vi "TDMSmanager.vi"(8 "ErrorIn":errorcluster, 11 "QueuesIn":T1) -> (0 "ErrorOut":errorcluster, 3 "QueuesOut":T1)   [LabVIEW 2019]
uses:
  utilities/AQueues.ctl
  AmasterVIs/ACommand.ctl
  analyzeAccelerationDataVIs/AccelerationDataFrames.ctl
  analyzeAccelerationDataVIs/AnalyzedVibrationsData.ctl
  analyzeAccelerationDataVIs/calculateFaultIndicatorsVIs/FaultDetections.ctl
  analyzeAccelerationDataVIs/calculateFaultIndicatorsVIs/ParameterFaultDetection.ctl
  analyzeAccelerationDataVIs/calculateFaultIndicatorsVIs/FaultParameter.ctl
  analyzeAccelerationDataVIs/calculateFaultIndicatorsVIs/FrequencyFaultDetection.ctl
  analyzeAccelerationDataVIs/calculateFaultIndicatorsVIs/OrdersFaultDetection.ctl
  TDMSmanagerVIs/TDMSAnalyzerData.ctl
  TDMSmanagerVIs/TDMSAnalyzerDataType.ctl
  TDMSmanagerVIs/TDMSmanagerState.ctl
  AmasterVIs/AThreads.ctl
  <vilib>/Platform/TimedLoop/XDataNode/timing_clust.ctl
  <vilib>/Platform/TimedLoop/XDataNode/nitl_modes.ctl
  <vilib>/Platform/TimedLoop/XDataNode/wakeup.ctl
  <vilib>/platform/TimedLoop/XDataNode/XDataNode.xnode
  <vilib>/Platform/TimedLoop/XDataNode/XDNodeRunTimeDep.lvlib
panel:
  in  "Restart":bool
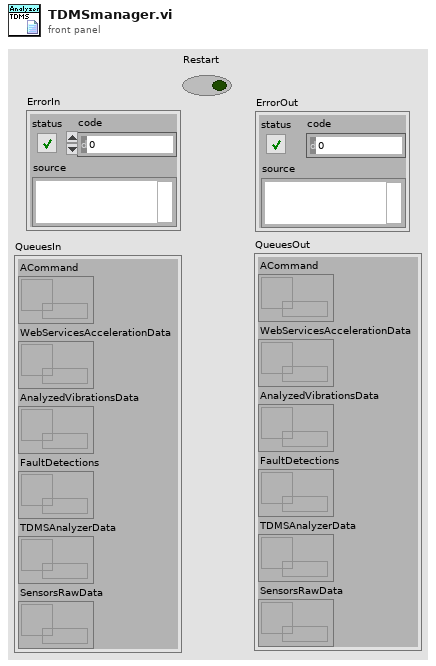
[diagram p1: front panel]
types:
  T1 = typedef "AQueues.ctl" = cluster{"ACommand":refnum<queue>, "WebServicesAccelerationData":refnum<queue>, "AnalyzedVibrationsData":refnum<queue>, "FaultDetections":refnum<queue>, "TDMSAnalyzerData":refnum<queue>, "SensorsRawData":refnum<queue>}
  T2 = typedef "AThreads.ctl" = enum16{"UI", "analyzeAccelerationData", "aquireAccelerationData", "communicateWebServices", "TDMSmanager", "aquireTachoSignal"}
  T3 = typedef "TDMSmanagerState.ctl" = enum16{"Idle", "SaveToFile", "SendFiles", "DeleteFiles", "CloseReference", "InitFileToSave"}
  T4 = typedef "XDNodeRunTimeDep.lvlib/timing_clust.ctl" = cluster{"Expected End [f-1]":u64, "Actual End [f-1]":u64, "Finished Late? [f-1]":bool, "Expected End [i-1]":u64, "Actual End [i-1]":u64, "Finished Late? [i-1]":bool, "Expected Start [i]":u64, "Actual Start [i]":u64, "Expected Start [f]":u64, "Actual Start [f]":u64, "Source Name":string, "Structure Name":string, "Period":i64, "Deadline":i64, "Offset":i64, "Start":i64, "Priority":i32, "Timeout":i32, "Mode":T5, "Wakeup Reason":T6, "Error":errorcluster, "Source Type":string, "Secondary Source Type":string, "Global End Time":u64, "Global Start Time":u64, "Frame Duration":u64, "Iteration Duration":u64, "Assigned CPU":i32, "I/O Scan Engine Mode":u32}
  T5 = typedef "XDNodeRunTimeDep.lvlib/nitl_modes.ctl" = enum32{"No Change", "Process missed periods, maintain original phase", "Discard missed periods, maintain original phase", "Process missed periods, ignore original phase", "Discard missed periods, ignore original phase"}
  T6 = typedef "XDNodeRunTimeDep.lvlib/wakeup.ctl" = enum32{"Normal", "Aborted", "Asynchronous wakeup", "Timing source error", "Timed loop error", "Timeout"}
  T7 = typedef "ACommand.ctl" = enum16{"None", "Start", "Stop", "Restart", "SendFilesData", "DeleteAllData"}
  T8 = enum16{"open", "replace", "create", "open or create", "replace or create", "replace or create with confirmation"}
  T9 = enum16{"open", "open or create", "create or replace", "create", "open (read-only)"}
  T10 = typedef "TDMSAnalyzerDataType.ctl" = enum16{"FileDataStart", "FileGroup", "FileDataStop", "NewFile", "EndOfFile"}
  T11 = typedef "TDMSAnalyzerData.ctl" = cluster{"TDMSAnalyzerDataType":T10, "group name out":string, "channel name(s) out":string[], "data":waveform(dbl)[], "File name":string}
  T12 = typedef "AnalyzerSettings.ctl" = cluster{"Create NS Timeout Code":i32, "Destroy NS Timeout Code":i32, "All threads":T2[], "AnalysisSettings":T13}
  T13 = typedef "AnalysisSettings.ctl" = cluster{"Fault Thresholds":T14, "Analysis series name":string, "Save data analysis?":bool, "Band size":i32, "OrderAnalysis?":bool, "Accelerometer":T16, "fs [Hz]":dbl, "Pulse per revolution":u16}
  T14 = typedef "Thresholds.ctl" = cluster{"Parameters labels":T15[], "Parameters thresholds":dbl[], "Freqs and thresholds":dbl[][], "Orders and thresholds":dbl[][]}
  T15 = typedef "FaultParameter.ctl" = enum16{"Kurtosis", "RMS", "Crest factor"}
  T16 = typedef "Accelerometer.ctl" = enum16{"None", "MPU6050", "MMA7351"}
  T17 = typedef "FaultDetections.ctl" = cluster{"Parameters fault detection":T18[], "Frequencies fault detection":T19[], "Orders fault detection":T20[]}
  T18 = typedef "ParameterFaultDetection.ctl" = cluster{"Axes Values":dbl[], "Axes Fault Detection":bool[], "Parameter Label":T15}
  T19 = typedef "FrequencyFaultDetection.ctl" = cluster{"Axes Values":dbl[], "Axes Fault Detection":bool[], "Frequency":dbl}
  T20 = typedef "OrdersFaultDetection.ctl" = cluster{"Order":dbl, "Axes Fault Detection":bool[], "Axes Values":dbl[]}
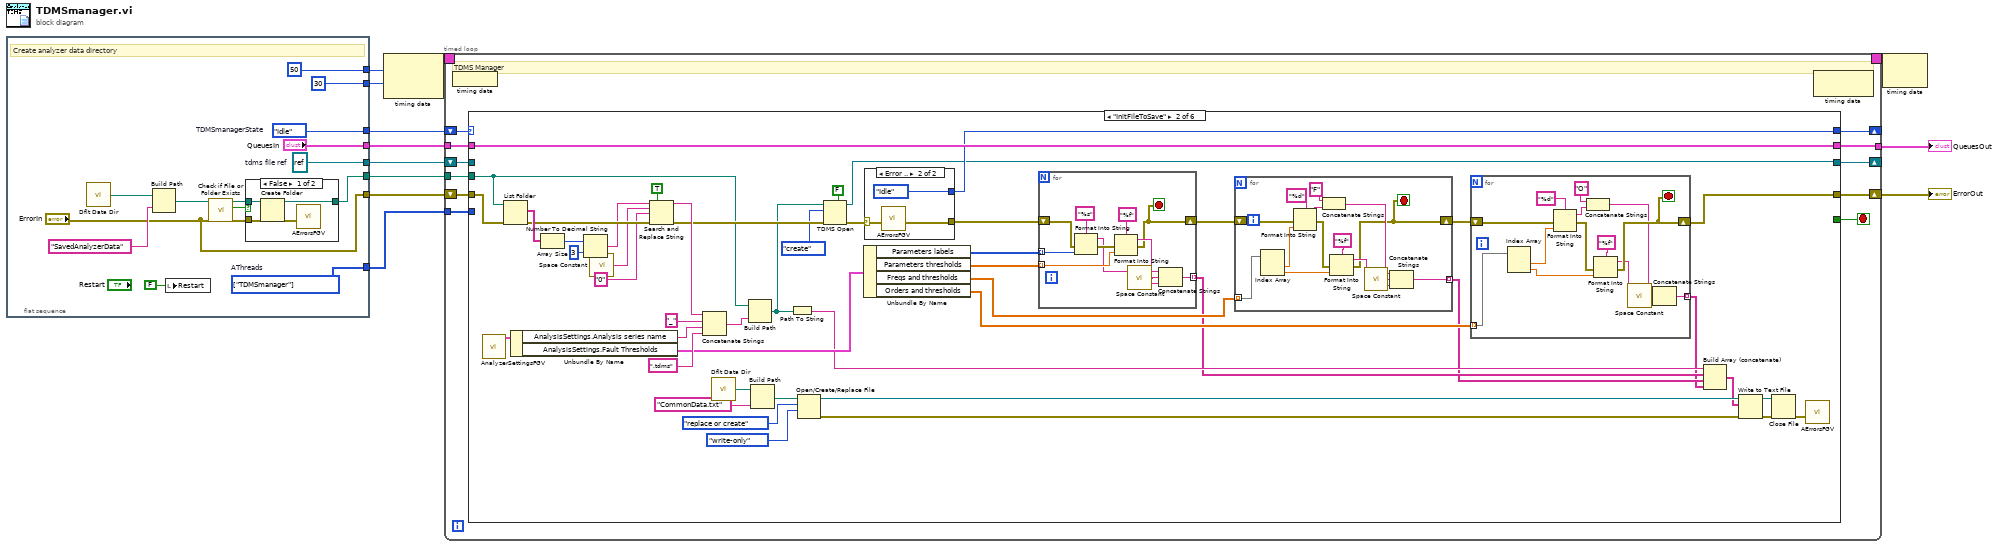
[diagram p0: block diagram]
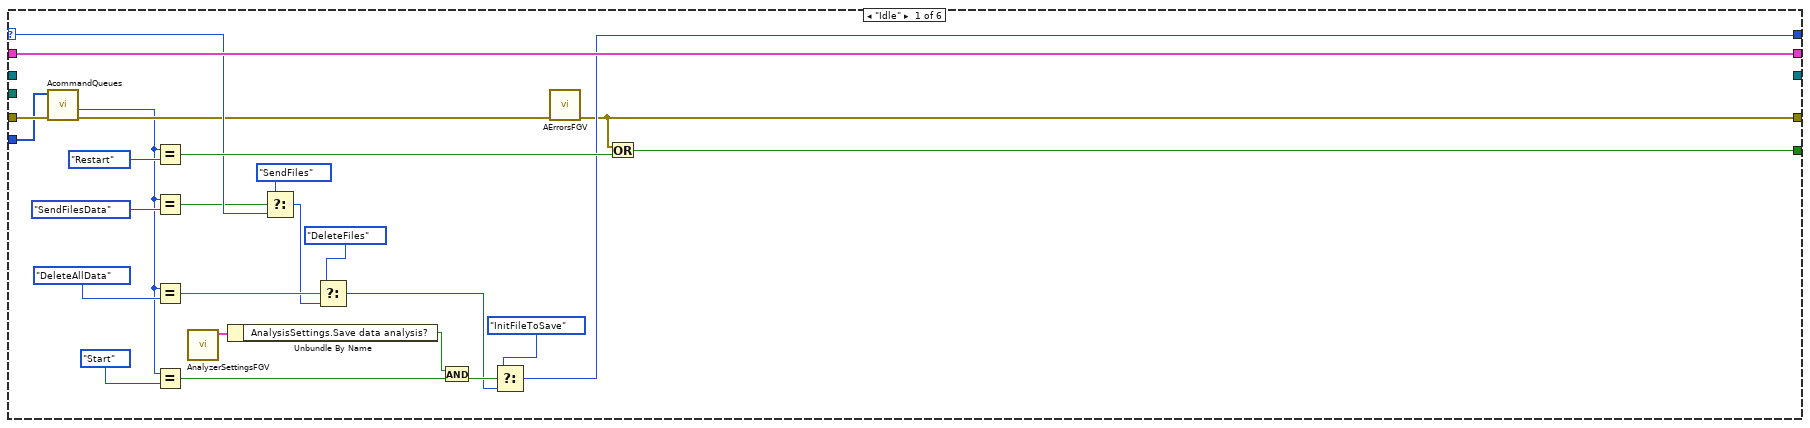
[diagram p2: hidden frame]
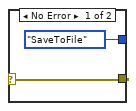
[diagram p3: hidden frame]
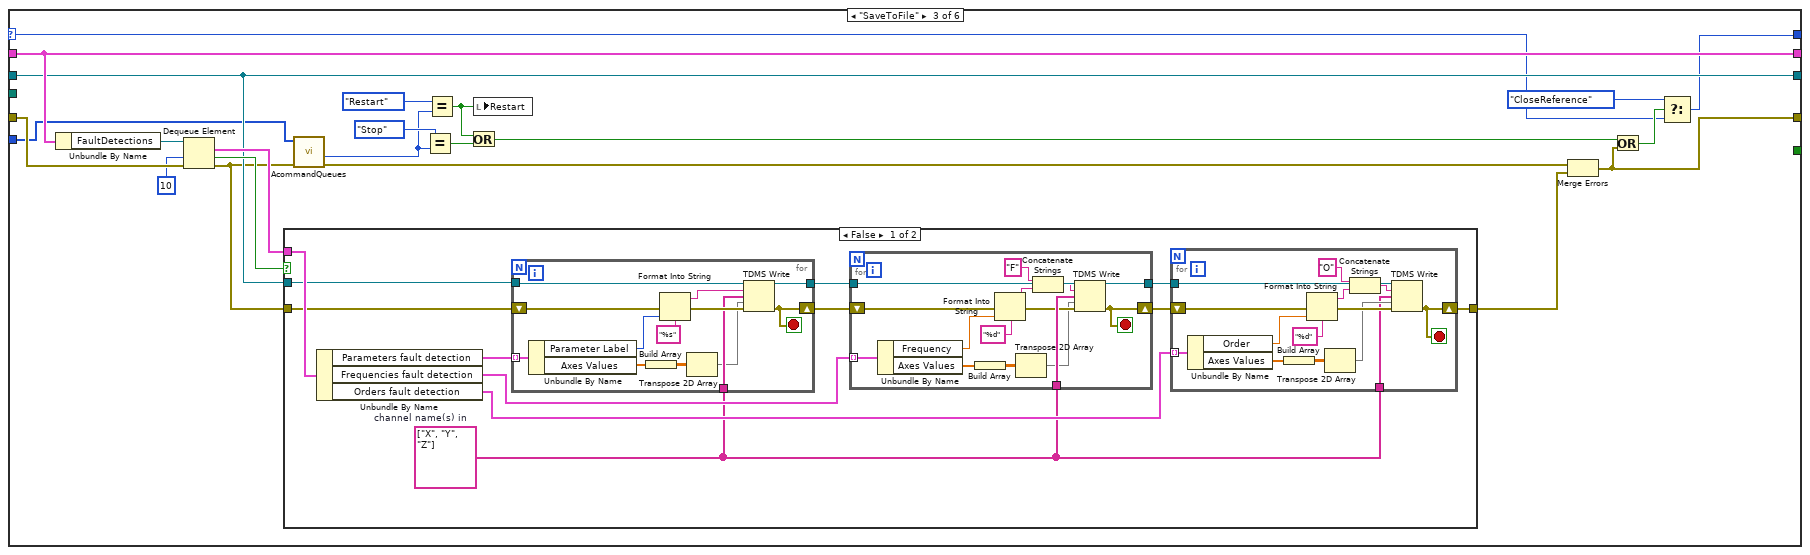
[diagram p4: hidden frame]
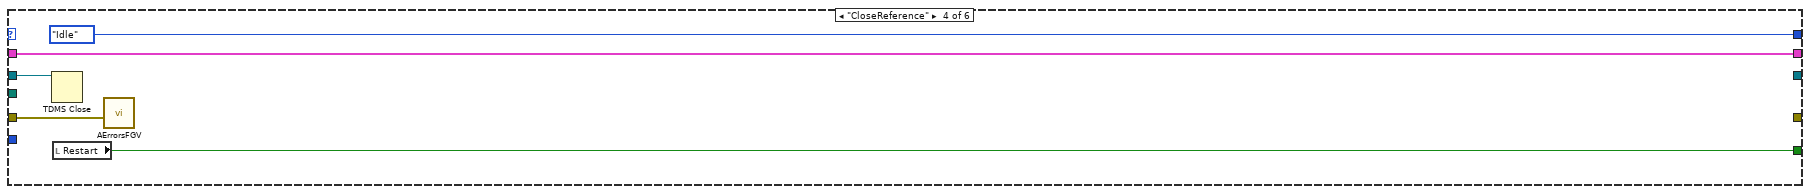
[diagram p6: hidden frame]
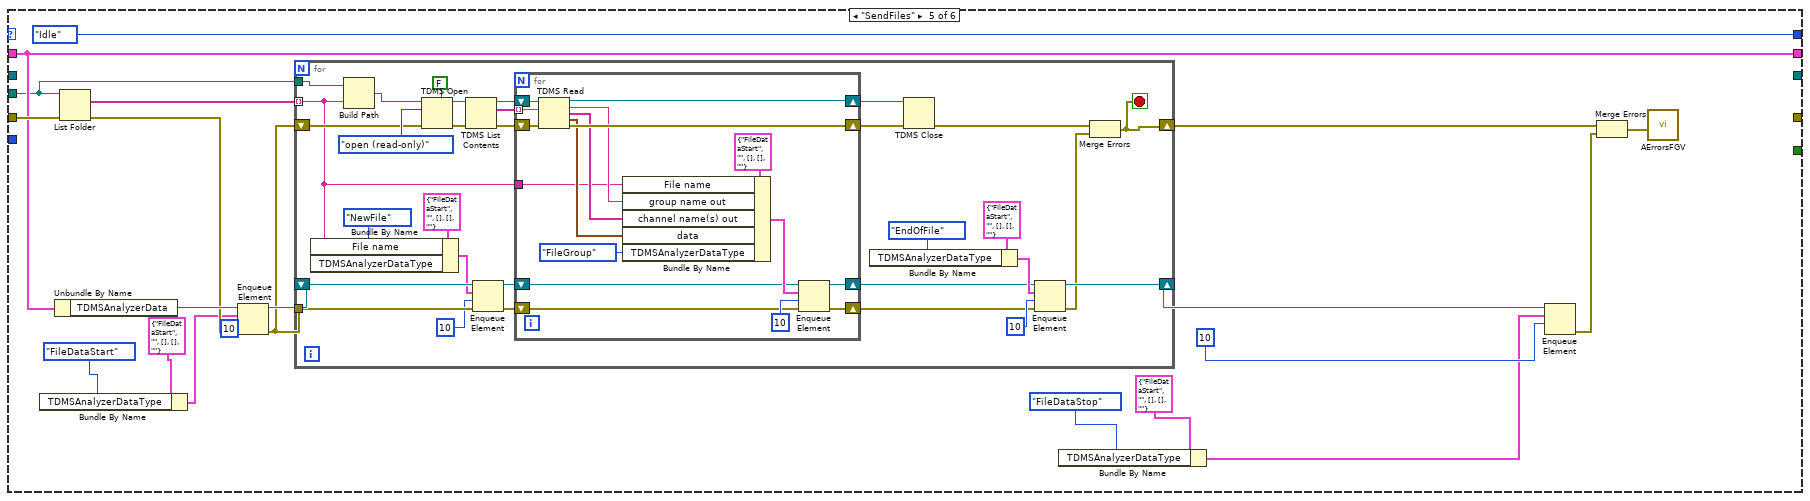
[diagram p7: hidden frame]
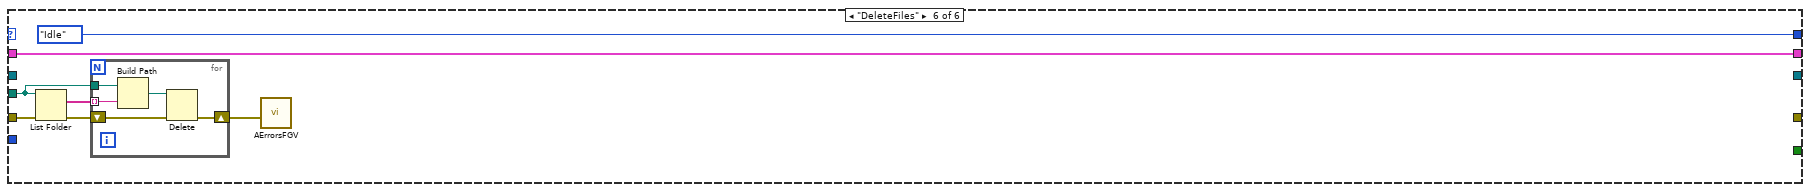
[diagram p8: hidden frame]
diagram:
  n1 = flat-sequence {
    tunnel: [w27] -> w12
    tunnel: ["QueuesIn"] -> w11
    tunnel: ["ErrorIn"] -> w8
    tunnel: [w20] -> w7
    tunnel: [w19] -> w6
    tunnel: [w17] -> w5
    tunnel: [i64 50 ("Period")] -> w2
    tunnel: [30 ("Priority")] -> w1
    frame #0 {
      w17 = T2[] [enum."TDMSmanager"] items=["UI", "analyzeAccelerationData", "aquireAccelerationData", "communicateWebServices", "TDMSmanager", "aquireTachoSignal"]  # AThreads
      w19 = refnum<k34> refnum  # tdms file ref
      w27 = TDMSmanagerState."Idle"  # TDMSmanagerState
      # "Create analyzer data directory"
      n2 = call <vilib>:"Dflt Data Dir.vi"() -> ("App:Default Data Directory"=w15:path)
      n3 = Build Path(base path=w15, name or relative path="SavedAnalyzerData") -> (appended path=w24:path)
      n4 = local write "Restart"(FALSE ("Restart")) -> ()
      n5 = call <vilib>:"Check if File or Folder Exists.vi"("error in (no error)"="ErrorIn", "path"=w24) -> ("error out"=w21:errorcluster, "file or folder exists?"=w23:bool, "dup path"=w22:path)  [unwired: 7 in]
      n6 = case shown="False" w23 {
        tunnel: w22 -> [w31 w32]
        tunnel: w21 -> [w28 _]
        tunnel: [w30 w32] -> w20
        frame False {
          n7 = Create Folder(path (use dialog)=w31, error in=w28) -> (created path=w30:path, error out=w29:errorcluster)  [unwired: 1 in, 1 out]
          n8 = call "AErrorsFGV.vi"("InternalErrorIn"=w29) -> ()  [unwired: 7 in, 4 out]
        }
        frame True {
        }
      }
    }
  }
  n9 = node-c288(w2, w1) -> (w4:T4)
  n10 = timed-loop {
    shift-right: [w40] -> _
    shift-left: w12 -> [w43]
    tunnel: w11 -> [w42]
    tunnel: [w41] -> w10
    shift-right: [w34] -> _
    shift-left: w6 -> [w36]
    shift-right: [w38] -> w9
    shift-left: w8 -> [w39]
    tunnel: w7 -> [w35]
    tunnel: w5 -> [w33]
    timing: w4 -> [_]
    timing-out: [_] -> w3
    stop <- w37 stop-if-true
    # "TDMS Manager"
    n11 = node-c288() -> ()  [unwired: 1 in]
    n12 = case shown="\"InitFileToSave\"" w43 {
      selector: w43 -> [w59 _ w169 _ _ _]
      tunnel: w42 -> [w70 w118 w184 w241 w255 w319]
      tunnel: [w70 w118 w184 w241 w255 w319] -> w41
      tunnel: [w53 w103 w167 TDMSmanagerState."Idle" ("TDMSmanagerState") TDMSmanagerState."Idle" ("TDMSmanagerState") TDMSmanagerState."Idle" ("TDMSmanagerState")] -> w40
      tunnel: w39 -> [w49 w117 w182 w243 w265 w317]
      tunnel: [w50 w79 w172 _ _ _] -> w38
      tunnel: [w51 _ _ w240 _ _] -> w37
      tunnel: w36 -> [_ _ w178 w244 _ _]
      tunnel: w35 -> [_ w97 _ _ w246 w314]
      tunnel: [_ w76 w178 _ _ _] -> w34
      tunnel: w33 -> [w48 _ w163 _ _ _]
      frame "Idle" {
        n13 = call "AcommandQueues.vi"("ErrorIn"=w49, "AThreads"=w48) -> ("ErrorOut"=w47:errorcluster, "ACommandOut"=w46:T7)  [unwired: 8 in]
        n14 = Equal?(x=w46, y=ACommand."Restart") -> (x = y?=w65:bool)
        n15 = Equal?(x=w46, y=ACommand."SendFilesData") -> (x = y?=w58:bool)
        n16 = Equal?(x=w46, y=ACommand."DeleteAllData") -> (x = y?=w55:bool)
        n17 = Equal?(x=w46, y=ACommand."Start") -> (x = y?=w63:bool)
        n18 = call "AnalyzerSettingsFGV.vi"() -> ("GlobalSettingsOut"=w64:T12)  [unwired: 11 in]
        n19 = Unbundle By Name(w64) -> ("AnalysisSettings.Save data analysis?"=w61:bool)
        n20 = Select(t=TDMSmanagerState."SendFiles", s=w58, f=w59) -> (s? t:f=w54:T3)
        n21 = Select(t=TDMSmanagerState."DeleteFiles", s=w55, f=w54) -> (s? t:f=w52:T3)
        n22 = And(x=w61, y=w63) -> (x .and. y?=w62:bool)
        n23 = Select(t=TDMSmanagerState."InitFileToSave", s=w62, f=w52) -> (s? t:f=w53:T3)
        n24 = call "AErrorsFGV.vi"("CriticalErrorIn"=w47) -> ("CriticalErrorOut"=w50:errorcluster)  [unwired: 7 in, 3 out]
        n25 = Or(x=w50, y=w65) -> (x .or. y?=w51:bool)
      }
      frame "InitFileToSave" {
        n26 = call "AnalyzerSettingsFGV.vi"() -> ("GlobalSettingsOut"=w102:T12)  [unwired: 11 in]
        n27 = List Folder(path=w97, error in=w117) -> (filenames=w116:string[], error out=w113:errorcluster)  [unwired: 2 in, 2 out]
        n28 = Unbundle By Name(w102) -> ("AnalysisSettings.Analysis series name"=w100:string, "AnalysisSettings.Fault Thresholds"=w85:T14)
        n29 = Array Size(array=w116) -> (size(s)=w115:i32)
        n30 = Number To Decimal String(number=w115, width (-)=i16 3) -> (decimal integer string=w112:string)
        n31 = call <vilib>:"Space Constant.vi"() -> ("String"=w110:string)
        n32 = Search and Replace String(replace all?=TRUE ("replace all? (F)"), input string=w112, search string=w110, replace string="0" ("replace string (\"\")"), error in=w113) -> (result string=w108:string, error out=w107:errorcluster)  [unwired: 3 in, 2 out]
        n33 = Concatenate Strings(w108, "_" ("string"), w100, ".tdms" ("string")) -> (w91:string)
        n34 = call <vilib>:"Dflt Data Dir.vi"() -> ("App:Default Data Directory"=w89:path)
        n35 = Build Path(base path=w97, name or relative path=w91) -> (appended path=w88:path)
        n36 = Build Path(base path=w89, name or relative path="CommonData.txt") -> (appended path=w96:path)
        n37 = Path To String(path=w88) -> (string=w75:string)
        n38 = Open/Create/Replace File(file path (use dialog)=w96, operation (0:open)=T8."replace or create", access (0:read/write)=enum16{"read/write", "read-only", "write-only"}."write-only") -> (refnum out=w93:refnum<file>, error out=w92:errorcluster)  [unwired: 3 in, 1 out]
        n39 = TDMS Open(5:FALSE ("create index file? (T)"), 8:w107, 10:T9."create" ("operation (0:open)"), 11:w88) -> (0:w104:errorcluster, 3:w76:refnum<k34>)  [unwired: 3 in]
        n40 = Unbundle By Name(w85) -> ("Parameters labels"=w87:T15[], "Parameters thresholds"=w86:dbl[], "Freqs and thresholds"=w82:dbl[][], "Orders and thresholds"=w80:dbl[][])
        n41 = case shown="Error .." w104 {
          selector: w104 -> [w158 w161]
          tunnel: [TDMSmanagerState."SaveToFile" ("TDMSmanagerState") TDMSmanagerState."Idle" ("TDMSmanagerState")] -> w103
          tunnel: [w158 w160] -> w84
          frame No Error {
          }
          frame Error {
            n42 = call "AErrorsFGV.vi"("InternalErrorIn"=w161) -> ("InternalErrorOut"=w160:errorcluster)  [unwired: 7 in, 3 out]
          }
        }
        n43 = for {
          tunnel: w87 -> [w156] mode=indexing
          tunnel: w86 -> [w154] mode=indexing
          shift-right: [w147] -> w83
          shift-left: w84 -> [w155]
          tunnel: [w148] -> w74 mode=indexing
          stop <- w147 stop-if-true
          n44 = Format Into String(format string="%s", error in=w155, w156) -> (resulting string=w151:string, error out=w153:errorcluster)  [unwired: 1 in]
          n45 = Format Into String(format string="%f", error in=w153, w154) -> (resulting string=w149:string, error out=w147:errorcluster)  [unwired: 1 in]
          n46 = call <vilib>:"Space Constant.vi"() -> ("String"=w150:string)
          n47 = Concatenate Strings(w151, w150, w149) -> (w148:string)
        }
        n48 = for {
          shift-right: [w133] -> w81
          shift-left: w83 -> [w146]
          tunnel: w82 -> [w142] mode=indexing
          tunnel: [w134] -> w73 mode=indexing
          stop <- w133 stop-if-true
          n49 = Index Array(array=w142) -> (element #1=w141:dbl, element #2=w139:dbl)  [unwired: 2 in]
          n50 = Format Into String(format string="%d", error in=w146, w141) -> (resulting string=w144:string, error out=w138:errorcluster)  [unwired: 1 in]
          n51 = Concatenate Strings("F" ("format string"), w144) -> (w136:string)
          n52 = Format Into String(format string="%f", error in=w138, w139) -> (resulting string=w135:string, error out=w133:errorcluster)  [unwired: 1 in]
          n53 = call <vilib>:"Space Constant.vi"() -> ("String"=w137:string)
          n54 = Concatenate Strings(w136, w137, w135) -> (w134:string)
        }
        n55 = for {
          shift-right: [w123] -> w79
          shift-left: w81 -> [w132]
          tunnel: w80 -> [w128] mode=indexing
          tunnel: [w119] -> w72 mode=indexing
          stop <- w123 stop-if-true
          n56 = Index Array(array=w128) -> (element #1=w127:dbl, element #2=w125:dbl)  [unwired: 2 in]
          n57 = Format Into String(format string="%d", error in=w132, w127) -> (resulting string=w130:string, error out=w124:errorcluster)  [unwired: 1 in]
          n58 = Concatenate Strings("O" ("format string"), w130) -> (w121:string)
          n59 = Format Into String(format string="%f", error in=w124, w125) -> (resulting string=w120:string, error out=w123:errorcluster)  [unwired: 1 in]
          n60 = call <vilib>:"Space Constant.vi"() -> ("String"=w122:string)
          n61 = Concatenate Strings(w121, w122, w120) -> (w119:string)
        }
        n62 = Build Array (concatenate)(w75, w74, w73, w72) -> (w71:string[])
        n63 = Write to Text File(file (use dialog)=w93, text=w71, error in=w92) -> (refnum out=w78:refnum<file>, error out=w77:errorcluster)  [unwired: 1 in, 1 out]
        n64 = Close File(refnum=w78, error in=w77) -> (error out=w90:errorcluster)  [unwired: 1 out]
        n65 = call "AErrorsFGV.vi"("InternalErrorIn"=w90) -> ()  [unwired: 7 in, 4 out]
      }
      frame "SaveToFile" {
        n66 = Unbundle By Name(w184) -> ("FaultDetections"=w183:refnum<queue>)
        n67 = Dequeue Element(queue=w183, timeout in ms (-1)=10, error in (no error)=w182) -> (element=w179:T17, timed out?=w180:bool, error out=w166:errorcluster)  [unwired: 1 out]
        n68 = case shown="False" w180 {
          tunnel: w179 -> [w196 _]
          tunnel: w178 -> [w194 _]
          tunnel: w166 -> [w195 w239]
          tunnel: [w188 w239] -> w173
          frame False {
            w186 = string[] ["X", "Y", "Z"]  # channel name(s) in
            n69 = Unbundle By Name(w196) -> ("Parameters fault detection"=w193:T18[], "Frequencies fault detection"=w191:T19[], "Orders fault detection"=w187:T20[])
            n70 = for {
              tunnel: w193 -> [w238] mode=indexing
              shift-right: [w231] -> w192
              shift-left: w195 -> [w237]
              tunnel: w194 -> [w234]
              tunnel: w186 -> [w230]
              tunnel: [w229] -> w190
              stop <- w231 stop-if-true
              n71 = Unbundle By Name(w238) -> ("Parameter Label"=w233:T15, "Axes Values"=w228:dbl[])
              n72 = Build Array(w228) -> (w227:dbl[][])
              n73 = Format Into String(format string="%s", error in=w237, w233) -> (resulting string=w232:string, error out=w235:errorcluster)  [unwired: 1 in]
              n74 = Transpose 2D Array(2D array=w227) -> (transposed array=w226:dbl[][])
              n75 = TDMS Write(0:w234, 5:w232, 7:w230, 9:w226, 11:w235) -> (4:w229:refnum<k34>, 15:w231:errorcluster)  [unwired: 1 in, 2 out]
            }
            n76 = for {
              tunnel: w191 -> [w225] mode=indexing
              shift-right: [w223] -> w189
              shift-left: w192 -> [w221]
              tunnel: w190 -> [w224]
              tunnel: w186 -> [w222]
              tunnel: [w214] -> w185
              stop <- w223 stop-if-true
              n77 = Unbundle By Name(w225) -> ("Frequency"=w220:dbl, "Axes Values"=w216:dbl[])
              n78 = Build Array(w216) -> (w217:dbl[][])
              n79 = Format Into String(format string="%d", error in=w221, w220) -> (resulting string=w212:string, error out=w218:errorcluster)  [unwired: 1 in]
              n80 = Transpose 2D Array(2D array=w217) -> (transposed array=w215:dbl[][])
              n81 = Concatenate Strings("F" ("format string"), w212) -> (w213:string)
              n82 = TDMS Write(0:w224, 5:w213, 7:w222, 9:w215, 11:w218) -> (4:w214:refnum<k34>, 15:w223:errorcluster)  [unwired: 1 in, 2 out]
            }
            n83 = for {
              shift-right: [w201] -> w188
              shift-left: w189 -> [w209]
              tunnel: w187 -> [w210] mode=indexing
              tunnel: w186 -> [w202]
              tunnel: w185 -> [w200]
              stop <- w201 stop-if-true
              n84 = Unbundle By Name(w210) -> ("Order"=w206:dbl, "Axes Values"=w204:dbl[])
              n85 = Build Array(w204) -> (w205:dbl[][])
              n86 = Format Into String(format string="%d", error in=w209, w206) -> (resulting string=w198:string, error out=w208:errorcluster)  [unwired: 1 in]
              n87 = Transpose 2D Array(2D array=w205) -> (transposed array=w203:dbl[][])
              n88 = Concatenate Strings("O" ("format string"), w198) -> (w199:string)
              n89 = TDMS Write(0:w200, 5:w199, 7:w202, 9:w203, 11:w208) -> (15:w201:errorcluster)  [unwired: 1 in, 3 out]
            }
          }
          frame True {
          }
        }
        n90 = call "AcommandQueues.vi"("ErrorIn"=w166, "AThreads"=w163) -> ("ErrorOut"=w165:errorcluster, "ACommandOut"=w164:T7)  [unwired: 8 in]
        n91 = Equal?(x=ACommand."Stop", y=w164) -> (x = y?=w175:bool)
        n92 = Equal?(x=ACommand."Restart", y=w164) -> (x = y?=w174:bool)
        n93 = Or(x=w174, y=w175) -> (x .or. y?=w171:bool)
        n94 = local write "Restart"(w174) -> ()
        n95 = Merge Errors(w165, w173) -> (w172:errorcluster)
        n96 = Or(x=w171, y=w172) -> (x .or. y?=w170:bool)
        n97 = Select(t=TDMSmanagerState."CloseReference", s=w170, f=w169) -> (s? t:f=w167:T3)
      }
      frame "CloseReference" {
        n98 = TDMS Close(11:w244) -> ()  [unwired: 1 in, 2 out]
        n99 = local read "Restart"() -> (w240:bool)
        n100 = call "AErrorsFGV.vi"("InternalErrorIn"=w243) -> ()  [unwired: 7 in, 4 out]
      }
      frame "SendFiles" {
        n101 = Bundle By Name(cluster=T11 {"TDMSAnalyzerDataType"=enum."FileDataStart", "group name out"="", "channel name(s) out"=[], "data"=[], "File name"=""} ("element"), "TDMSAnalyzerDataType"=TDMSAnalyzerDataType."FileDataStart") -> (w251:T11)
        n102 = Unbundle By Name(w255) -> ("TDMSAnalyzerData"=w261:refnum<queue>)
        n103 = List Folder(path=w246, error in=w265) -> (filenames=w247:string[], error out=w260:errorcluster)  [unwired: 2 in, 2 out]
        n104 = Enqueue Element(queue=w261, element=w251, timeout in ms (-1)=10, error in (no error)=w260) -> (queue out=w262:refnum<queue>, error out=w245:errorcluster)  [unwired: 1 out]
        n105 = for {
          shift-right: [w288] -> w257
          shift-left: w245 -> [w295]
          tunnel: w247 -> [w266] mode=indexing
          tunnel: w246 -> [w290]
          tunnel: w245 -> [w280]
          shift-right: [w268] -> w259
          shift-left: w262 -> [w282]
          stop <- w288 stop-if-true
          n106 = Bundle By Name(cluster=T11 {"TDMSAnalyzerDataType"=enum."FileDataStart", "group name out"="", "channel name(s) out"=[], "data"=[], "File name"=""} ("element"), "File name"=w266, "TDMSAnalyzerDataType"=TDMSAnalyzerDataType."NewFile") -> (w277:T11)
          n107 = Build Path(base path=w290, name or relative path=w266) -> (appended path=w289:path)
          n108 = TDMS Open(5:FALSE ("create index file? (T)"), 8:w295, 10:T9."open (read-only)" ("operation (0:open)"), 11:w289) -> (0:w286:errorcluster, 3:w287:refnum<k34>)  [unwired: 3 in]
          n109 = TDMS List Contents(4:w286, 7:w287) -> (0:w284:errorcluster, 2:w283:string[], 3:w285:refnum<k34>)  [unwired: 1 in, 1 out]
          n110 = Enqueue Element(queue=w282, element=w277, timeout in ms (-1)=10, error in (no error)=w280) -> (queue out=w281:refnum<queue>, error out=w279:errorcluster)  [unwired: 1 out]
          n111 = for {
            tunnel: w266 -> [w299]
            shift-right: [w310] -> w292
            shift-left: w285 -> [w313]
            shift-right: [w311] -> w293
            shift-left: w284 -> [w312]
            shift-right: [w303] -> w270
            shift-left: w281 -> [w305]
            tunnel: w283 -> [w298] mode=indexing
            shift-right: [w304] -> w269
            shift-left: w279 -> [w297]
            n112 = TDMS Read(0:w313, 5:w298, 11:w312) -> (4:w310:refnum<k34>, 6:w302:string, 8:w300:string[], 10:w301:waveform(dbl)[], 15:w311:errorcluster)  [unwired: 5 in, 1 out]
            n113 = Bundle By Name(cluster=T11 {"TDMSAnalyzerDataType"=enum."FileDataStart", "group name out"="", "channel name(s) out"=[], "data"=[], "File name"=""} ("element"), "File name"=w299, "group name out"=w302, "channel name(s) out"=w300, "data"=w301, "TDMSAnalyzerDataType"=TDMSAnalyzerDataType."FileGroup") -> (w307:T11)
            n114 = Enqueue Element(queue=w305, element=w307, timeout in ms (-1)=10, error in (no error)=w297) -> (queue out=w303:refnum<queue>, error out=w304:errorcluster)  [unwired: 1 out]
          }
          n115 = Bundle By Name(cluster=T11 {"TDMSAnalyzerDataType"=enum."FileDataStart", "group name out"="", "channel name(s) out"=[], "data"=[], "File name"=""} ("element"), "TDMSAnalyzerDataType"=TDMSAnalyzerDataType."EndOfFile") -> (w274:T11)
          n116 = TDMS Close(8:w293, 11:w292) -> (0:w291:errorcluster)  [unwired: 1 out]
          n117 = Enqueue Element(queue=w270, element=w274, timeout in ms (-1)=10, error in (no error)=w269) -> (queue out=w268:refnum<queue>, error out=w267:errorcluster)  [unwired: 1 out]
          n118 = Merge Errors(w291, w267) -> (w288:errorcluster)
        }
        n119 = Bundle By Name(cluster=T11 {"TDMSAnalyzerDataType"=enum."FileDataStart", "group name out"="", "channel name(s) out"=[], "data"=[], "File name"=""} ("element"), "TDMSAnalyzerDataType"=TDMSAnalyzerDataType."FileDataStop") -> (w248:T11)
        n120 = Enqueue Element(queue=w259, element=w248, timeout in ms (-1)=10) -> (error out=w256:errorcluster)  [unwired: 1 in, 2 out]
        n121 = Merge Errors(w257, w256) -> (w254:errorcluster)
        n122 = call "AErrorsFGV.vi"("InternalErrorIn"=w254) -> ()  [unwired: 7 in, 4 out]
      }
      frame "DeleteFiles" {
        n123 = List Folder(path=w314, error in=w317) -> (filenames=w315:string[], error out=w316:errorcluster)  [unwired: 2 in, 2 out]
        n124 = for {
          tunnel: w315 -> [w324] mode=indexing
          tunnel: w314 -> [w323]
          shift-right: [w325] -> w318
          shift-left: w316 -> [w322]
          n125 = Build Path(base path=w323, name or relative path=w324) -> (appended path=w321:path)
          n126 = Delete(path (use dialog)=w321, error in=w322) -> (error out=w325:errorcluster)  [unwired: 3 in, 2 out]
        }
        n127 = call "AErrorsFGV.vi"("InternalErrorIn"=w318) -> ()  [unwired: 7 in, 4 out]
      }
    }
    n128 = node-c288() -> ()  [unwired: 1 in, 1 out]
  }
  "ErrorOut" <- w9
  "QueuesOut" <- w10
  n129 = node-c288(w3) -> ()  [unwired: 1 out]
